vi "OpenMainDB.vi"() -> (0 "头信息":string)   [LabVIEW 2014]
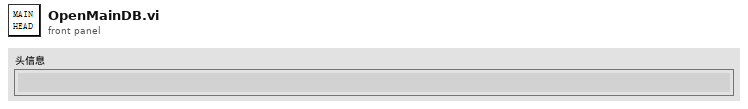
[diagram p1: front panel]
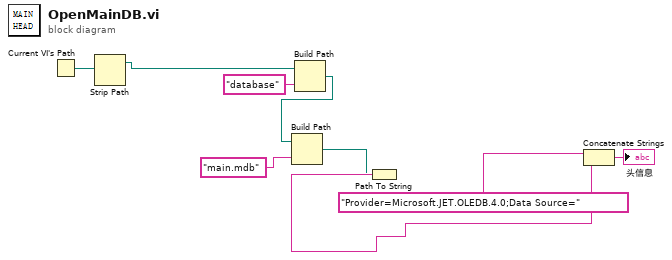
[diagram p0: block diagram]
diagram:
  n1 = Current VI's Path() -> (path=w5:path)
  n2 = Strip Path(path=w5) -> (stripped path=w6:path)  [unwired: 1 out]
  n3 = Build Path(base path=w6, name or relative path="database" ("名称或相对路径")) -> (appended path=w3:path)
  n4 = Build Path(base path=w3, name or relative path="main.mdb" ("名称或相对路径")) -> (appended path=w2:path)
  n5 = Path To String(path=w2) -> (string=w9:string)
  n6 = Concatenate Strings("Provider=Microsoft.JET.OLEDB.4.0;Data Source=", w9) -> (→"头信息":string)
